vi "Modulo de adquisición (SubVI).vi"(11 "file path (use dialog)":path) -> (0 "error out":errorcluster, 2 "error out 2":errorcluster)   [LabVIEW 2023]
panel:
  out "subarray":dbl[](array[numeric])
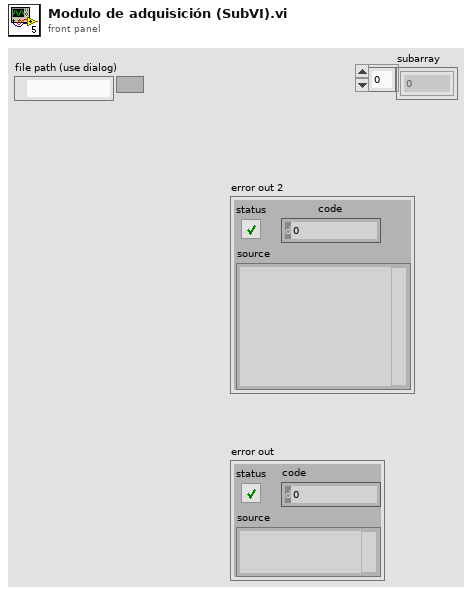
[diagram p1: front panel]
types:
  T1 = enum16{"open", "replace", "create", "open or create", "replace or create", "replace or create with confirmation"}
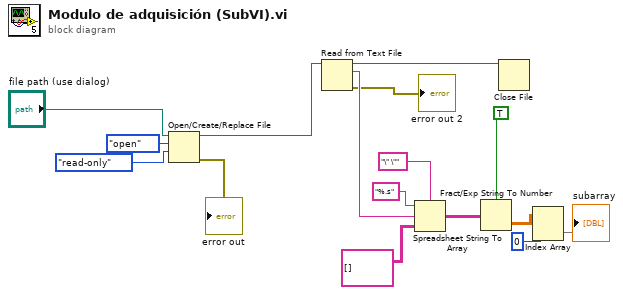
[diagram p0: block diagram]
diagram:
  n1 = Open/Create/Replace File(file path (use dialog)="file path (use dialog)", operation (0:open)=T1."open", access (0:read/write)=enum16{"read/write", "read-only", "write-only"}."read-only") -> (refnum out=w7:refnum<file>, error out=→"error out":errorcluster)  [unwired: 3 in, 1 out]
  n2 = Read from Text File(file (use dialog)=w7) -> (refnum out=w8:refnum<file>, text=w12:string, error out=→"error out 2":errorcluster)  [unwired: 3 in, 1 out]
  n3 = Spreadsheet String To Array(delimiter (Tab)="\" \"", format string="%.s", spreadsheet string=w12, array type (2D Dbl)=string[][] []) -> (array=w14:string[][])
  n4 = Fract/Exp String To Number(use system decimal point (T)=TRUE, string=w14) -> (number=w3:dbl[][])  [unwired: 2 in, 1 out]
  n5 = Close File(refnum=w8) -> ()  [unwired: 1 in, 2 out]
  n6 = Index Array(array=w3, index (col)=0 ("disabled index (col)")) -> (element=→"subarray":dbl[])  [unwired: 1 in]
